vi "test Endpoint Configurations.vi"(8 "error in (no error)":errorcluster, 11 "TestCase in":refnum<class "NI-SWITCH Scripting Unit Tests.lvclass">) -> (0 "error out":errorcluster, 3 "TestCase out":refnum<class "NI-SWITCH Scripting Unit Tests.lvclass">)   [LabVIEW 2017, in "NI-SWITCH Scripting Unit Tests.lvclass"]
uses:
  NI-SWITCH Scripting Unit Tests.lvclass
  <vilib>/addons/_JKI Toolkits/VI Tester/TestCase.llb/TestCase.lvclass
  NI-SWITCH Scripting.lvlib
  Shared/Endpoint Configuration Enum.ctl
  Shared/NI-SWITCH Shared.lvlib
  Shared/Endpoint Configuration Cluster.ctl
  Custom Device/Find All SLSC Switch Custom Devices.vi
  <vilib>/NI Veristand/Custom Device API/Custom Device Item Ref.ctl
  <vilib>/NI VeriStand/Custom Device API/Custom Device API.lvlib
  Shared/Routing and Faulting Hardware API/Routing and Faulting Hardware API.lvlib
  C:/Program Files (x86)/National Instruments/LabVIEW 2017/vi.lib/addons/_JKI Toolkits/VI Tester/TestCase.llb/TestCase.lvclass
panel:
  in  "Save?":bool
  out "Output Filename":string
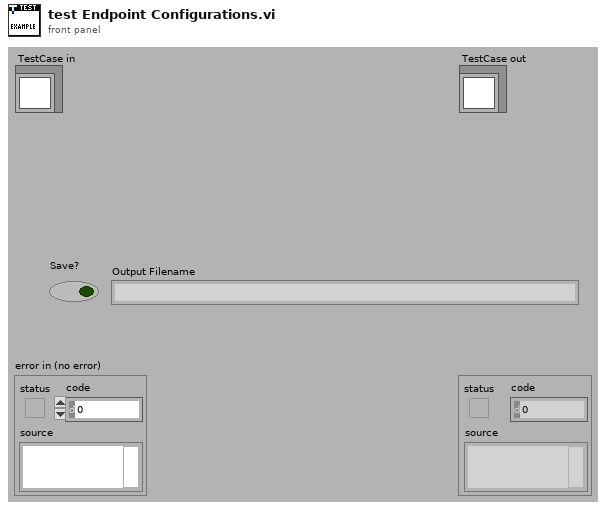
[diagram p1: front panel]
types:
  T1 = typedef "Custom Device API.lvlib/Custom Device Item Ref.ctl" = u64
  T2 = typedef "NI-SWITCH Shared.lvlib/Endpoint Configuration Cluster.ctl" = cluster{"Endpoint":string, "Configuration":T3}
  T3 = typedef "NI-SWITCH Shared.lvlib/Endpoint Configuration Enum.ctl" = enum16{"Load", "Source", "Configuration"}
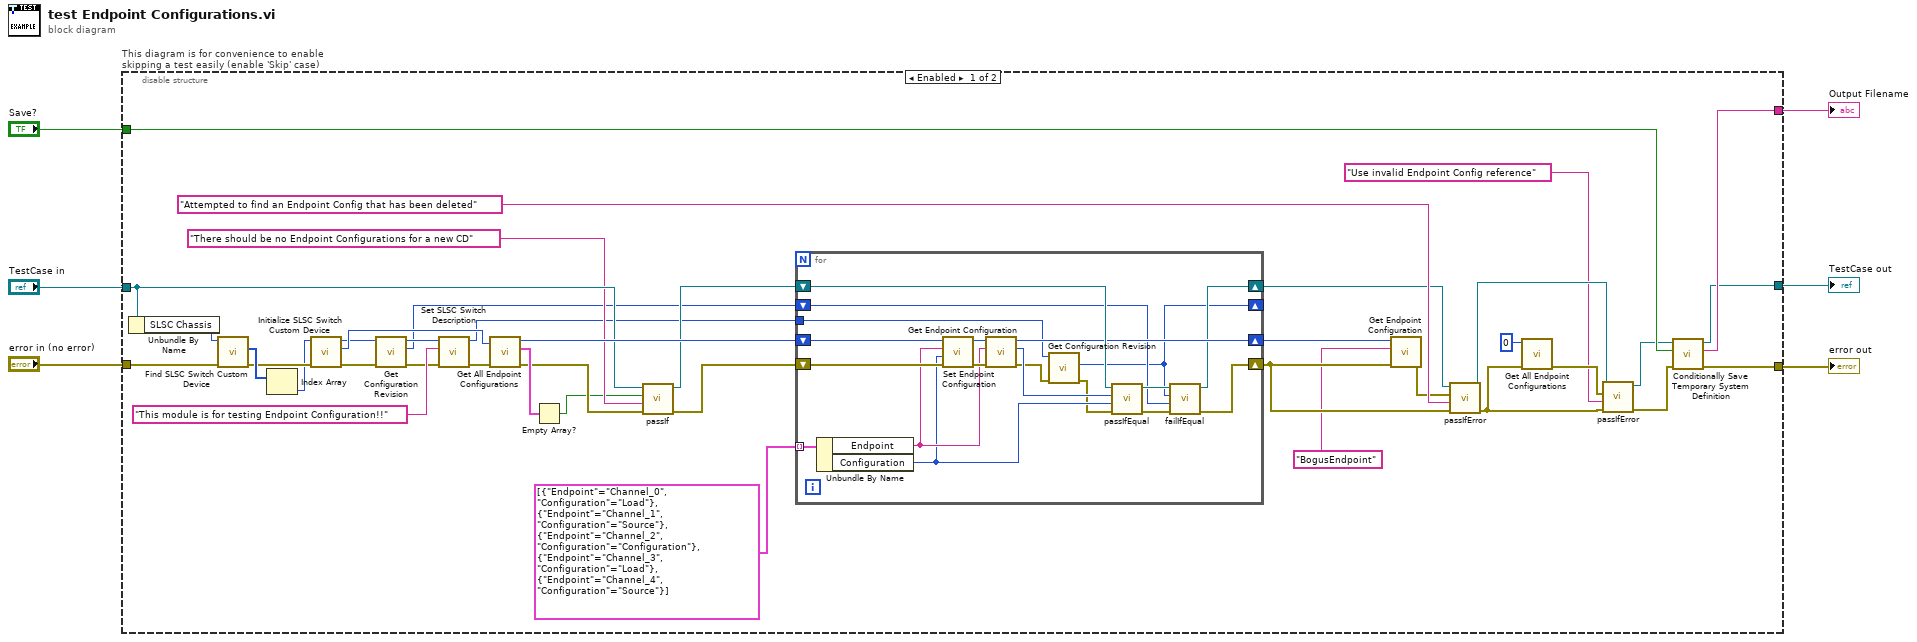
[diagram p0: block diagram]
diagram:
  n1 = disable-structure "This diagram is for convenience to enable skipping a test easily (enable 'Skip' case)" shown="Enabled" {
    disable-tunnel: "TestCase in" -> [w33 w69]
    disable-tunnel: [w44 w67] -> w3
    disable-tunnel: [w45 w68] -> w5
    disable-tunnel: "error in (no error)" -> [w38 w66]
    disable-tunnel: [w46 _] -> w2
    disable-tunnel: "Save?" -> [w43 _]
    frame Enabled {
      n2 = Unbundle By Name(w33) -> ("SLSC Chassis"=w39:u64)
      n3 = call-poly "Find SLSC Switch Custom Device.vi"("error in"=w38, "slsc chassis in"=w39) -> ("error out"=w41:errorcluster, "slsc switch custom devices"=w42:T1[])  [unwired: 7 in, 1 out]
      n4 = Index Array(array=w42) -> (element=w40:T1)  [unwired: 1 in]
      n5 = call "Initialize SLSC Switch Custom Device.vi"("error in"=w41, "slsc switch custom device in"=w40) -> ("error out"=w10:errorcluster, "endpoint configuration section"=w36:T1, "slsc switch custom device out"=w12:T1)  [unwired: 7 in]
      n6 = call "Get Configuration Revision.vi"("error in (no error)"=w10, "Hardware Ref in"=w12) -> ("error out"=w9:errorcluster, "Configuration Revision"=w7:u32, "Hardware Ref out"=w11:T1)  [unwired: 6 in, 1 out]
      n7 = call "Set SLSC Switch Description.vi"("error in"=w9, "description"="This module is for testing Endpoint Configuration!!" ("Description"), "slsc switch custom device in"=w11) -> ("error out"=w29:errorcluster, "slsc switch custom device out"=w8:T1)  [unwired: 7 in]
      n8 = call "Get All Endpoint Configurations.vi"("error in"=w29, "endpoint configuration in"=w36) -> ("error out"=w23:errorcluster, "endpoint configurations"=w34:T2[], "endpoint configuration out"=w35:T1)  [unwired: 7 in]
      n9 = Empty Array?(array=w34) -> (empty?=w21:bool)
      n10 = call-dynamic "passIf.vi"("error in (no error)"=w23, "message (\"\")"="There should be no Endpoint Configurations for a new CD" ("message (\"\")"), "pass"=w21, "TestCase in"=w33) -> ("error out"=w30:errorcluster, "TestCase out"=w32:refnum<class "NI-SWITCH Scripting Unit Tests.lvclass">)  [unwired: 6 in]
      n11 = for {
        shift-right: [w51] -> w27
        shift-left: w30 -> [w64]
        shift-right: [w49] -> w25
        shift-left: w32 -> [w61]
        shift-right: [w59] -> w28
        shift-left: w35 -> [w65]
        tunnel: T2[] [{"Endpoint"="Channel_0", "Configuration"=enum."Load"}, {"Endpoint"="Channel_1", "Configuration"=enum."Source"}, {"Endpoint"="Channel_2", "Configuration"=enum."Configuration"}, {"Endpoint"="Channel_3", "Configuration"=enum."Load"}, {"Endpoint"="Channel_4", "Configuration"=enum."Source"}] ("Array") -> [w57] mode=indexing
        tunnel: w8 -> [w52]
        shift-right: [w47] -> _
        shift-left: w7 -> [w48]
        n12 = Unbundle By Name(w57) -> ("Endpoint"=w56:string, "Configuration"=w55:T3)
        n13 = call "Set Endpoint Configuration.vi"("error in"=w64, "configuration"=w55, "endpoint"=w56, "endpoint configuration in"=w65) -> ("error out"=w62:errorcluster, "endpoint configuration out"=w63:T1)  [unwired: 6 in]
        n14 = call "Get Endpoint Configuration.vi"("error in"=w62, "endpoint"=w56, "endpoint configuration in"=w63) -> ("error out"=w54:errorcluster, "configuration"=w58:T3, "endpoint configuration out"=w59:T1)  [unwired: 6 in]
        n15 = call "Get Configuration Revision.vi"("error in (no error)"=w54, "Hardware Ref in"=w52) -> ("error out"=w53:errorcluster, "Configuration Revision"=w47:u32)  [unwired: 6 in, 2 out]
        n16 = call-dynamic "passIfEqual.vi"("error in (no error)"=w53, "y"=w55, "x"=w58, "TestCase in"=w61) -> ("error out"=w60:errorcluster, "TestCase out"=w50:refnum<class "NI-SWITCH Scripting Unit Tests.lvclass">)  [unwired: 6 in]
        n17 = call-dynamic "failIfEqual.vi"("error in (no error)"=w60, "y"=w48, "x"=w47, "TestCase in"=w50) -> ("error out"=w51:errorcluster, "TestCase out"=w49:refnum<class "NI-SWITCH Scripting Unit Tests.lvclass">)  [unwired: 6 in]
      }
      n18 = call "Get Endpoint Configuration.vi"("error in"=w27, "endpoint"="BogusEndpoint" ("Endpoint"), "endpoint configuration in"=w28) -> ("error out"=w24:errorcluster)  [unwired: 6 in, 2 out]
      n19 = call-dynamic "passIfError.vi"("error in (no error)"=w27, "task (\"\")"="Attempted to find an Endpoint Config that has been deleted" ("message (\"\")"), "error"=w24, "TestCase in"=w25) -> ("error out"=w13:errorcluster, "TestCase out"=w18:refnum<class "NI-SWITCH Scripting Unit Tests.lvclass">)  [unwired: 6 in]
      n20 = call "Get All Endpoint Configurations.vi"("error in"=w13, "endpoint configuration in"=T1 0 ("Endpoint Configuration Section Ref in")) -> ("error out"=w15:errorcluster)  [unwired: 7 in, 2 out]
      n21 = call-dynamic "passIfError.vi"("error in (no error)"=w13, "task (\"\")"="Use invalid Endpoint Config reference" ("message (\"\")"), "error"=w15, "TestCase in"=w18) -> ("error out"=w19:errorcluster, "TestCase out"=w17:refnum<class "NI-SWITCH Scripting Unit Tests.lvclass">)  [unwired: 6 in]
      n22 = call "Conditionally Save Temporary System Definition.vi"("error in (no error)"=w19, "Save?"=w43, "Test Case"=w17) -> ("error out"=w45:errorcluster, "filename"=w46:string, "Test Case"=w44:refnum<class "NI-SWITCH Scripting Unit Tests.lvclass">)  [unwired: 6 in]
    }
    frame Disabled {
      # "skip test result while test is under development"
      n23 = call <vilib>:"skip.vi"("error in (no error)"=w66, "TestCase in"=w69) -> ("error out"=w68:errorcluster, "TestCase out"=w67:refnum<class "NI-SWITCH Scripting Unit Tests.lvclass">)  [unwired: 8 in]
    }
  }
  "error out" <- w5
  "TestCase out" <- w3
  "Output Filename" <- w2
